vi "Initialize.vi"(8 "error in (no error)":errorcluster, 11 "User Interface in":refnum<class "User Interface.lvclass">) -> (0 "error out":errorcluster, 3 "User Interface out":refnum<class "User Interface.lvclass">)   [LabVIEW 2019, in "DSF Core.lvlib" / "User Interface.lvclass"]
uses:
  User Interface.lvclass
  User Interface.lvclass/User Interface.ctl
  User Interface Events/User Interface Events.lvclass
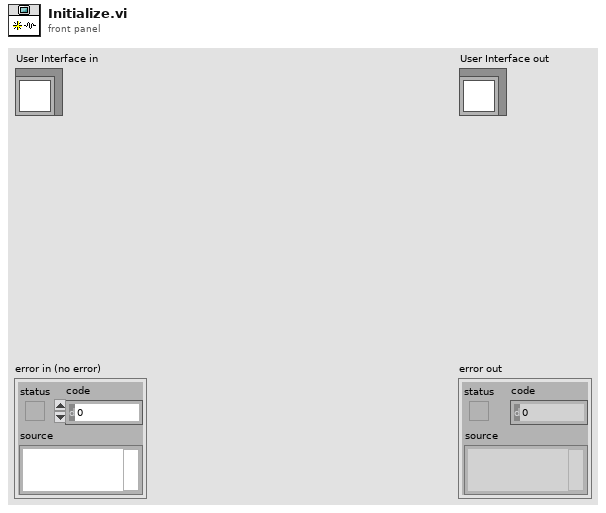
[diagram p1: front panel]
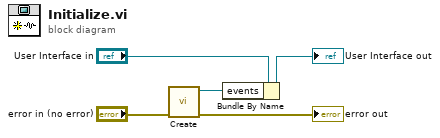
[diagram p0: block diagram]
diagram:
  n1 = call "Create.vi"("error in (no error)"="error in (no error)") -> ("error out"=→"error out":errorcluster, "User Interface Events out"=w4:refnum<class "User Interface Events.lvclass">)  [unwired: 9 in]
  n2 = Bundle By Name(cluster="User Interface in", "events"=w4) -> (→"User Interface out":refnum<class "User Interface.lvclass">)
